vi "SW_Generate_Segmented_Plot_v2.vi"(0 "Draw Area Size":cluster{"Width":dbl, "Height":dbl}={"Width"=480.0, "Height"=480.0}, 1 "Input cluster of parameters":T1={"Amount of border segments"=8, "Border segments starting angle"=0, "Amount of midfield segments"=4, "Midfield segments starting angle"=0, "Midfield segments outer radius, mm"=60, "Amount of central segments"=1, "Center segment outer radius, mm"=30}, 2 "Diameter of the cage, mm":u16(knob)=180 scale=20.0..250.0, 3 "R-gap between segments, mm":u8=10, 4 "Colors array for outer segments":u32[](array[numeric])=[14102567, 16625249, 14742520, 7646673, 16018755, 16703632, 11262441, 4552116], 5 "Error In":errorcluster, 6 "Regions to mark":u16[](array[numeric]), 7 "Colors array for midfield segments":u32[](array[numeric])=[8073876, 10935200, 34871, 12756431], 9 "Color for central segment":u32=16777113) -> (12 "No zones Display output":picture, 14 "Zones Display output":picture, 15 "Actual parameters output":T4, 16 "Array of the segment to color correspondences":u32[][](array[numeric]), 17 "Array of the pixel to color correspondences":u32[][](array[numeric]), 18 "Pixels per mm":dbl=2.533333333333333, 19 "Error Out":errorcluster)   [LabVIEW 2018]
panel:
  out "Fonts scale factor":dbl
  out "Coordinates of the center of the image":T2
  out "Center segments outer radius, pix":dbl
  out "Midfield segments outer radius, pix":dbl
  out "Bounding rectangle of the midfield segments":T3
  out "Bounding rectangle for outer segments":T3
  in  "Fill color for no segments image":u32(colorbox)=6316128
  out "Radius of displayed outer segments, pix":dbl=228.0
  in  "Background color":u32(colorbox)=13816530
  in  "Zones Display input":picture
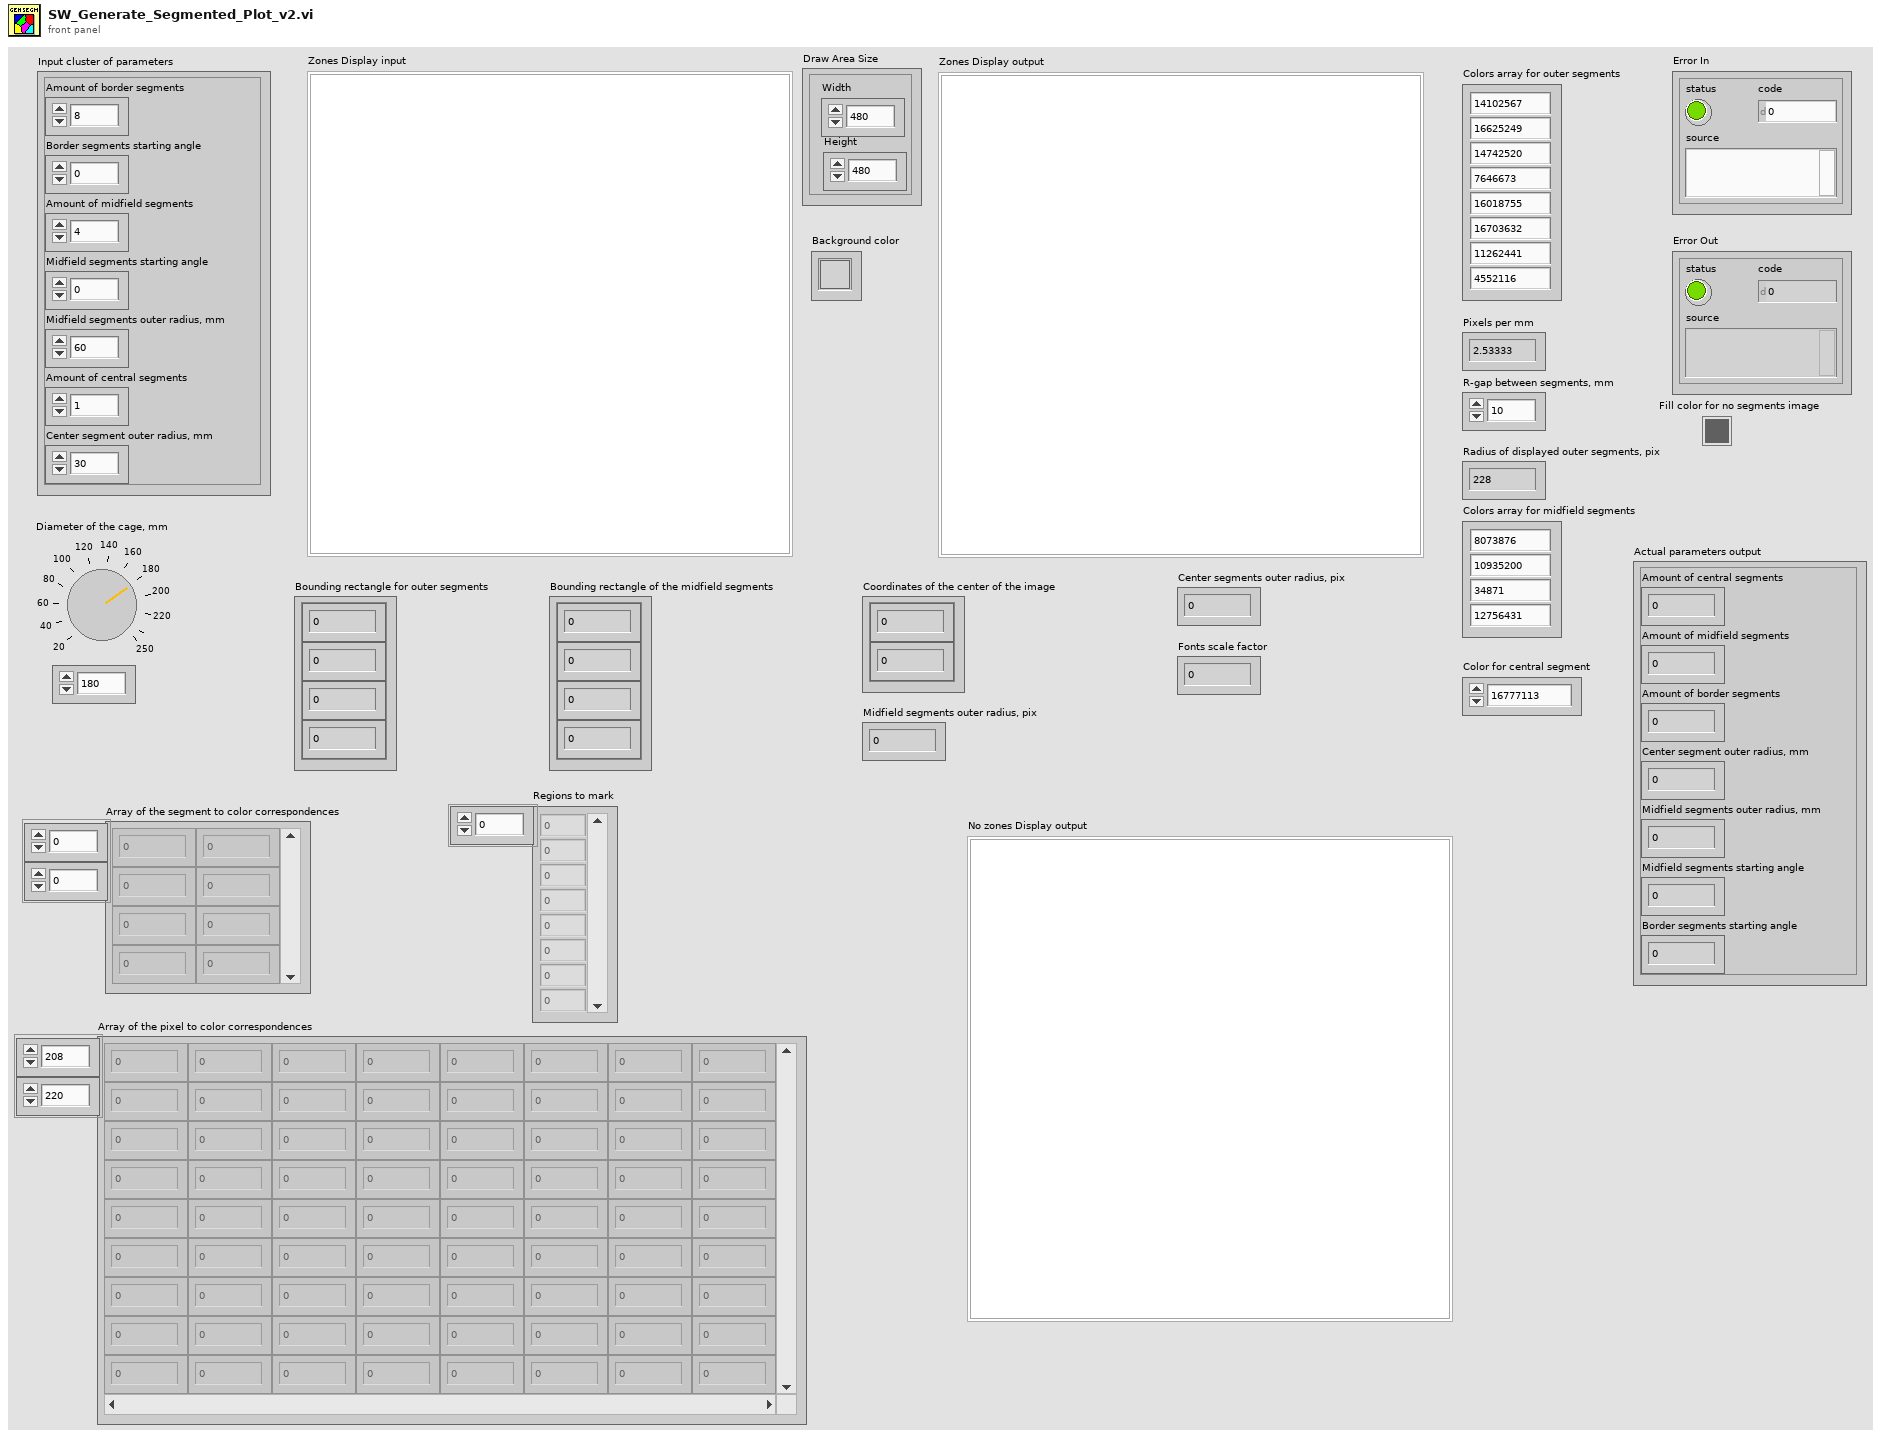
[diagram p1: front panel]
types:
  T1 = cluster{"Amount of border segments":u8, "Border segments starting angle":i16, "Amount of midfield segments":u8, "Midfield segments starting angle":i16, "Midfield segments outer radius, mm":u16, "Amount of central segments":u8, "Center segment outer radius, mm":u16}
  T2 = cluster{"Numeric Control":dbl, "Numeric Control":dbl}
  T3 = cluster{"Numeric Control":dbl, "Numeric Control":dbl, "Numeric Control":dbl, "Numeric Control":dbl}
  T4 = cluster{"Amount of central segments":u8, "Amount of midfield segments":u8, "Amount of border segments":u8, "Center segment outer radius, mm":u16, "Midfield segments outer radius, mm":u16, "Midfield segments starting angle":i16, "Border segments starting angle":i16}
  T5 = enum16{"User-specified Font", "Application Font", "System Font", "Dialog Font"}
  T6 = cluster{"horizontal":enum16{"left", "center", "right"}, "vertical":enum16{"top", "center", "bottom"}}
  T7 = cluster{"Width":u16, "Style":enum32{"Solid", "Dash", "Dot", "DashDot", "DashDotDot"}}
  T8 = cluster{"Amount of central segments":u8, "Amount of midfield segments":u8, "Amount of border segments":u8, u16, u16, i16, i16}
  T9 = typedef "imagedata.ctl" = cluster{"image type":i32, "image depth":i32, "image":u8[], "mask":u8[], "colors":u32[], "Rectangle":cluster{"left":i16, "top":i16, "right":i16, "bottom":i16}}
  T10 = cluster{"left":i16, "top":i16, "right":i16, "bottom":i16}
  T11 = cluster{"image[0]":u8, "image[1]":u8, "image[2]":u8}
  T12 = cluster{"Font Name:":string, "Size":i16, "Strikeout?":bool, "Italic?":bool, "Underline?":bool, "Outline?":bool, "Shadow?":bool, "Bold?":bool}
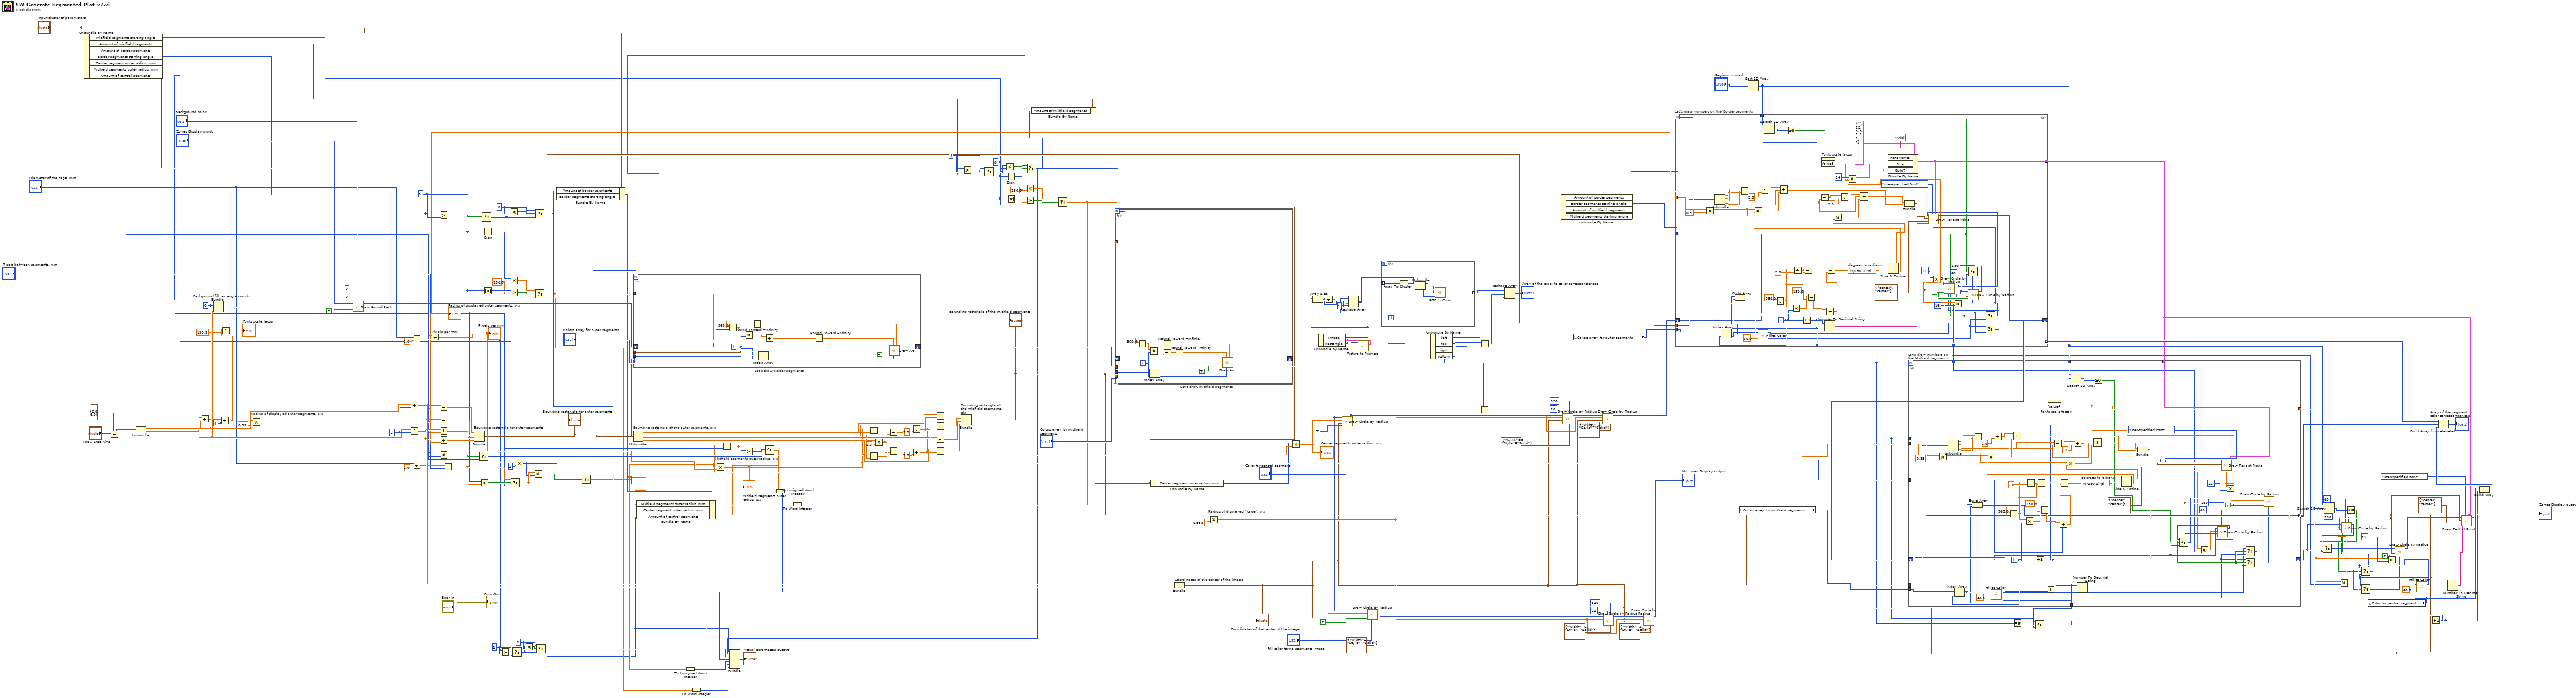
[diagram p0: block diagram]
diagram:
  w66 = 3 ("dimension size")
  w14 = TRUE ("fill?(F)")
  w150 = 180.0 ("y")
  w156 = u8 1 ("y")
  w153 = u8 1 ("y")
  w157 = u8 4 ("y")
  w160 = u8 0 ("y")
  w180 = u8 0 ("y")
  w182 = u8 8 ("y")
  w185 = 180.0 ("y")
  w194 = u32 2 ("y")
  w196 = 0
  n1 = Unbundle By Name("Input cluster of parameters") -> ("Midfield segments starting angle"=w37:i16, "Amount of midfield segments"=w36:u8, "Amount of border segments"=w35:u8, "Border segments starting angle"=w34:i16, "Center segment outer radius, mm"=w33:u16, "Midfield segments outer radius, mm"=w32:u16, "Amount of central segments"=w31:u8)
  n2 = Subtract(x="Draw Area Size", y=cluster{"Width":dbl, "Height":dbl} {"Width"=6.0, "Height"=6.0}) -> (x-y=w91:cluster{"Width":dbl, "Height":dbl})
  n3 = Unbundle(w91) -> ("Width"=w192:dbl, "Height"=w193:dbl)
  n4 = Add(x=w193, y=w192) -> (x+y=w191:dbl)
  n5 = Bundle "Background fill rectangle coords"(w196, w196, "Width"=w192, "Height"=w193) -> (w178:cluster{i32, i32, "Width":dbl, "Height":dbl})  [unwired: 1 in]
  n6 = Divide(x=w191, y=u32 4) -> (x/y=w30:dbl)
  n7 = Divide(x=w30, y=199.5) -> (x/y=→"Fonts scale factor":dbl)
  n8 = Multiply "Radius of displayed outer segments, pix"(x=w30, y=0.95) -> (x*y=w78:dbl)
  "Radius of displayed outer segments, pix" <- w78
  n9 = call <vilib>:"Draw Round Rect.vi"("picture"="Zones Display input", "oval width"=i16 0, "rect"=w178, "fill?(F)"=TRUE, "color(black)"="Background color", "oval height"=i16 0) -> ("new picture"=w177:picture)  [unwired: 3 in]
  n10 = Divide(x=w192, y=w194) -> (x/y=w176:dbl)
  n11 = Divide(x=w193, y=w194) -> (x/y=w175:dbl)
  n12 = Divide(x="Diameter of the cage, mm", y=2.0) -> (x/y=w164:dbl)
  n13 = Divide(x="Diameter of the cage, mm", y=2.0) -> (x/y=w142:dbl)
  n14 = Divide "Pixels per mm"(x=w78, y=w164) -> (x/y=w104:dbl)
  "Pixels per mm" <- w104
  n15 = Greater?(x=w35, y=w182) -> (0:w183:bool)
  n16 = Subtract(x=w176, y=w78) -> (x-y=w174:dbl)
  n17 = Subtract(x=w175, y=w78) -> (x-y=w173:dbl)
  n18 = Add(x=w176, y=w78) -> (x+y=w172:dbl)
  n19 = Add(x=w175, y=w78) -> (x+y=w171:dbl)
  n20 = Less?(x=w33, y="R-gap between segments, mm") -> (x < y?=w140:bool)
  n21 = Subtract(x=w142, y="R-gap between segments, mm") -> (x-y=w145:dbl)
  n22 = Bundle "Bounding rectangle for outer segments"(w174, w173, w172, w171) -> (w79:cluster{dbl, dbl, dbl, dbl})  [unwired: 1 in]
  "Bounding rectangle for outer segments" <- w79
  n23 = Select(t="R-gap between segments, mm", s=w140, f=w33) -> (s? t:f=w137:u16)
  n24 = Greater?(x=w32, y=w145) -> (0:w146:bool)
  n25 = Select(t=w182, s=w183, f=w35) -> (s? t:f=w179:u8)
  n26 = Sign(1:w34) -> (0:w186:i16)
  n27 = Absolute Value(x=w34) -> (abs(x)=w188:i16)
  n28 = Greater?(x=w31, y=w156) -> (0:w155:bool)
  n29 = Less?(x=w179, y=w180) -> (x < y?=w181:bool)
  n30 = Multiply(x=w186, y=w185) -> (x*y=w184:dbl)
  n31 = Greater?(x=w188, y=w185) -> (0:w187:bool)
  n32 = Select(t=w145, s=w146, f=w32) -> (s? t:f=w143:dbl)
  n33 = Select(t=w156, s=w155, f=w31) -> (s? t:f=w152:u8)
  n34 = Multiply(x="R-gap between segments, mm", y=u8 2) -> (x*y=w136:u8)
  n35 = Less?(x=w152, y=w153) -> (x < y?=w154:bool)
  n36 = Less?(x=w143, y=w136) -> (x < y?=w144:bool)
  n37 = Select(t=w180, s=w181, f=w179) -> (s? t:f=w51:u8)
  n38 = Select(t=w184, s=w187, f=w34) -> (s? t:f=w50:dbl)
  n39 = Select(t=w153, s=w154, f=w152) -> (s? t:f=w44:u8)
  n40 = Bundle By Name(cluster="Input cluster of parameters", "Amount of border segments"=w51, "Border segments starting angle"=w50) -> (w48:T1)
  n41 = Select(t=w136, s=w144, f=w143) -> (s? t:f=w46:dbl)
  n42 = for "Let's draw border segments" {
    N: w51 -> [w207]
    tunnel: w50 -> [w212]
    shift-right: [w205] -> w162
    shift-left: w177 -> [w214]
    tunnel: w79 -> [w208]
    tunnel: "Colors array for outer segments" -> [w211]
    i -> [w202]
    n43 = Divide(x=360.0, y=w207) -> (x/y=w206:dbl)
    n44 = Multiply(x=w206, y=w202) -> (x*y=w213:dbl)
    n45 = Round Toward +Infinity(x=w206) -> (ceil(x): smallest int >= x=w204:dbl)
    n46 = Index Array(array=w211, index=w202) -> (element=w201:u32)
    n47 = Add(x=w213, y=w212) -> (x+y=w209:dbl)
    n48 = Round Toward -Infinity(1:w209) -> (0:w203:dbl)
    n49 = call <vilib>:"Draw Arc.vi"("picture"=w214, "start angle[degrees]"=w203, "rect"=w208, "fill?(F)"=TRUE, "color(black)"=w201, "arc size[degrees]"=w204) -> ("new picture"=w205:picture)  [unwired: 3 in]
  }
  n50 = Unbundle "Bounding rectangle of the outer segments, pix"(w79) -> (w130:dbl, w122:dbl, w128:dbl, w121:dbl)
  n51 = To Unsigned Word Integer(number=w46) -> (unsigned 16bit integer=w109:u16)
  n52 = To Word Integer(number=w50) -> (16bit integer=w105:i16)
  n53 = Multiply "Midfield segments outer radius, pix"(x=w46, y=w104) -> (x*y=w76:dbl)
  "Midfield segments outer radius, pix" <- w76
  n54 = Subtract(x=w46, y="R-gap between segments, mm") -> (x-y=w138:dbl)
  n55 = Greater?(x=w137, y=w138) -> (0:w139:bool)
  n56 = Select(t=w138, s=w139, f=w137) -> (s? t:f=w45:dbl)
  n57 = Bundle By Name(cluster=w48, "Midfield segments outer radius, mm"=w46, "Center segment outer radius, mm"=w45, "Amount of central segments"=w44) -> (w47:T1)
  n58 = To Unsigned Word Integer(number=w45) -> (unsigned 16bit integer=w107:u16)
  n59 = Subtract(x=w128, y=w130) -> (x-y=w134:dbl)
  n60 = Subtract(x=w121, y=w122) -> (x-y=w127:dbl)
  n61 = Multiply(x=w76, y=2.0) -> (x*y=w126:dbl)
  n62 = Subtract(x=w134, y=w126) -> (x-y=w132:dbl)
  n63 = Subtract(x=w127, y=w126) -> (x-y=w124:dbl)
  n64 = Divide(x=w132, y=2.0) -> (x/y=w129:dbl)
  n65 = Divide(x=w124, y=2.0) -> (x/y=w123:dbl)
  n66 = Add(x=w130, y=w129) -> (x+y=w120:dbl)
  n67 = Add(x=w122, y=w123) -> (x+y=w118:dbl)
  n68 = Subtract(x=w128, y=w129) -> (x-y=w119:dbl)
  n69 = Subtract(x=w121, y=w123) -> (x-y=w117:dbl)
  n70 = Bundle "Bounding rectangle of the midfield segments, pix"(w120, w118, w119, w117) -> (w77:cluster{dbl, dbl, dbl, dbl})  [unwired: 1 in]
  "Bounding rectangle of the midfield segments" <- w77
  n71 = Greater?(x=w36, y=w157) -> (0:w158:bool)
  n72 = Select(t=w157, s=w158, f=w36) -> (s? t:f=w161:u8)
  n73 = Less?(x=w161, y=w160) -> (x < y?=w159:bool)
  n74 = Sign(1:w37) -> (0:w149:i16)
  n75 = Absolute Value(x=w37) -> (abs(x)=w147:i16)
  n76 = Multiply(x=w149, y=w150) -> (x*y=w151:dbl)
  n77 = Greater?(x=w147, y=w150) -> (0:w148:bool)
  n78 = Select(t=w160, s=w159, f=w161) -> (s? t:f=w49:u8)
  n79 = Bundle By Name(cluster=w47, "Amount of midfield segments"=w49) -> (w42:T1)
  n80 = Select(t=w151, s=w148, f=w37) -> (s? t:f=w108:dbl)
  n81 = To Word Integer(number=w108) -> (16bit integer=w106:i16)
  n82 = Bundle("Amount of central segments"=w44, "Amount of midfield segments"=w49, "Amount of border segments"=w51, w107, w109, w106, w105) -> (→"Actual parameters output":T8)  [unwired: 1 in]
  n83 = for "Let's draw midfield segments" {
    N: w49 -> [w221]
    shift-right: [w216] -> w97
    shift-left: w162 -> [w217]
    tunnel: w108 -> [w219]
    tunnel: w46 -> [_]
    tunnel: w77 -> [w218]
    tunnel: "Colors array for midfield segments" -> [w223]
    i -> [w220]
    n84 = Divide(x=360.0, y=w221) -> (x/y=w225:dbl)
    n85 = Multiply(x=w225, y=w220) -> (x*y=w226:dbl)
    n86 = Index Array(array=w223, index=w220) -> (element=w222:u32)
    n87 = Round Toward +Infinity(x=w225) -> (ceil(x): smallest int >= x=w228:dbl)
    n88 = Add(x=w226, y=w219) -> (x+y=w227:dbl)
    n89 = Round Toward -Infinity(1:w227) -> (0:w229:dbl)
    n90 = call <vilib>:"Draw Arc.vi"("picture"=w217, "start angle[degrees]"=w229, "rect"=w218, "fill?(F)"=TRUE, "color(black)"=w222, "arc size[degrees]"=w228) -> ("new picture"=w216:picture)  [unwired: 3 in]
  }
  n91 = Unbundle By Name(w42) -> ("Center segment outer radius, mm"=w43:u16)
  n92 = Bundle "Coordinates of the center of the image"(w176, w175) -> (w17:cluster{dbl, dbl})  [unwired: 1 in]
  "Coordinates of the center of the image" <- w17
  n93 = Multiply "Radius of displayed \"cage\", pix"(x=w30, y=0.955) -> (x*y=w93:dbl)
  n94 = Multiply(x=w43, y=w104) -> (x*y=w113:dbl)
  "Center segments outer radius, pix" <- w113
  n95 = call <vilib>:"Draw Circle by Radius.vi"("color(black)"="Color for central segment", "fill?(F)"=TRUE, "pixel center"=w17, "radius"=w113, "picture"=w97) -> ("new picture"=w70:picture)  [unwired: 6 in]
  n96 = call <vilib>:"Picture to Pixmap.vi"("picture"=w70) -> ("image data"=w69:T9)  [unwired: 9 in, 1 out]
  n97 = Unbundle By Name(w69) -> ("image"=w68:u8[], "Rectangle"=w63:T10)
  n98 = Array Size(array=w68) -> (size(s)=w67:i32)
  n99 = Divide(x=w67, y=w66) -> (x/y=w65:dbl)
  n100 = Reshape Array(w68, w65, w66) -> (w64:u8[][])
  n101 = call <vilib>:"Draw Circle by Radius.vi"("pen"=T7 {"Width"=2, "Style"=enum."Solid"}, "color(black)"="Fill color for no segments image", "fill?(F)"=TRUE, "pixel center"=w17, "radius"=w93, "picture"=w97) -> ("new picture"=w94:picture)  [unwired: 5 in]
  n102 = for {
    tunnel: w64 -> [w236] mode=indexing
    tunnel: [w231] -> w62 mode=indexing
    n103 = Array To Cluster(array=w236) -> (cluster=w235:T11)
    n104 = Unbundle(w235) -> ("image[0]"=w234:u8, "image[1]"=w233:u8, "image[2]"=w232:u8)
    n105 = call <vilib>:"RGB to Color.vi"("B"=w232, "G"=w233, "R"=w234) -> ("Color"=w231:u32)
  }
  n106 = Unbundle By Name(w63) -> ("left"=w60:i16, "top"=w57:i16, "right"=w61:i16, "bottom"=w58:i16)
  n107 = Subtract(x=w58, y=w57) -> (x-y=w56:i16)
  n108 = Subtract(x=w61, y=w60) -> (x-y=w59:i16)
  n109 = Reshape Array(w62, w59, w56) -> (→"Array of the pixel to color correspondences":u32[][])
  n110 = Unbundle By Name(w42) -> ("Amount of border segments"=w41:u8, "Border segments starting angle"=w40:i16, "Amount of midfield segments"=w5:u8, "Midfield segments starting angle"=w39:i16)
  n111 = call <vilib>:"Draw Circle by Radius.vi"("pen"=T7 {"Width"=6, "Style"=enum."Solid"}, "arc size(360)"=i16 320, "start angle(0)"=i16 20, "pixel center"=w17, "radius"=w93, "picture"=w70) -> ("new picture"=w170:picture)  [unwired: 5 in]
  n112 = local read "Colors array for outer segments"() -> (w86:u32[])
  n113 = call <vilib>:"Draw Circle by Radius.vi"("pen"=T7 {"Width"=2, "Style"=enum."Solid"}, "pixel center"=w17, "radius"=w93, "picture"=w170) -> ("new picture"=w88:picture)  [unwired: 7 in]
  n114 = call <vilib>:"Draw Circle by Radius.vi"("pen"=T7 {"Width"=6, "Style"=enum."Solid"}, "arc size(360)"=i16 320, "start angle(0)"=i16 20, "pixel center"=w17, "radius"=w93, "picture"=w94) -> ("new picture"=w98:picture)  [unwired: 5 in]
  n115 = call <vilib>:"Draw Circle by Radius.vi"("pen"=T7 {"Width"=2, "Style"=enum."Solid"}, "pixel center"=w17, "radius"=w93, "picture"=w98) -> ("new picture"=→"No zones Display output":picture)  [unwired: 7 in]
  n116 = local read "Colors array for midfield segments"() -> (w85:u32[])
  n117 = Sort 1D Array(array="Regions to mark") -> (sorted array=w21:u16[])
  n118 = for "Let's draw numbers on the Border segments" {
    N: w41 -> [w303]
    tunnel: w40 -> [w304]
    shift-right: [w283] -> w87
    shift-left: w88 -> [w246]
    tunnel: w79 -> [w298]
    tunnel: w86 -> [w271]
    tunnel: w78 -> [w268]
    tunnel: [w255] -> w2
    tunnel: [w265] -> w74 mode=indexing
    tunnel: [w257] -> w27
    tunnel: w21 -> [w256]
    tunnel: [w242] -> w1
    i -> [w270]
    w242 = 16 ("y")
    w251 = TRUE ("fill?(F)")
    n119 = Multiply(x=w268, y=0.9) -> (x*y=w267:dbl)
    n120 = Unbundle(w298) -> (w292:dbl, w285:dbl, w297:dbl, w284:dbl)
    n121 = Index Array(array=w271, index=w270) -> (element=w243:u32)
    n122 = Subtract(x=w297, y=w292) -> (x-y=w295:dbl)
    n123 = call <vilib>:"Hilite Color.vi"("Percentage(30)"=60.0, "Color In"=w243) -> ("Shadow"=w241:u32, "Hilite"=w240:u32)
    n124 = Divide(x=w295, y=2.0) -> (x/y=w293:dbl)
    n125 = Divide(x=360.0, y=w303) -> (x/y=w273:dbl)
    n126 = Multiply(x=w273, y=w270) -> (x*y=w277:dbl)
    n127 = Divide(x=w273, y=2.0) -> (x/y=w275:dbl)
    n128 = Increment(x=w270) -> (x+1=w255:i32)
    n129 = Build Array(w243, w255) -> (w265:u32[])
    n130 = Search 1D Array(1D array=w256, element=w255) -> (index of element=w254:i32)  [unwired: 1 in]
    n131 = Greater Or Equal To 0?(x=w254) -> (x >= 0?=w239:bool)
    n132 = Subtract(x=w275, y=w273) -> (x-y=w274:dbl)
    n133 = Subtract(x=w277, y=180.0) -> (x-y=w278:dbl)
    n134 = Subtract(x=w284, y=w285) -> (x-y=w287:dbl)
    n135 = property on="Fonts scale factor" class="DigNum (strict)"() -> ("Value"=w250:dbl)  [unwired: 2 in, 2 out]
    n136 = Number To Decimal String(number=w255) -> (decimal integer string=w281:string)  [unwired: 1 in]
    n137 = Add(x=w278, y=w304) -> (x+y=w301:dbl)
    n138 = Subtract(x=w274, y=w301) -> (x-y=w300:dbl)
    n139 = Divide(x=w287, y=2.0) -> (x/y=w289:dbl)
    n140 = Multiply(x=i16 14 ("Size"), y=w250) -> (x*y=w259:dbl)
    n141 = expression code="(x/180.0)*pi" "degrees to radians"(w300) -> (w299:dbl)
    n142 = Bundle By Name(cluster=T12 {"Font Name:"="", "Size"=12, "Strikeout?"=FALSE, "Italic?"=FALSE, "Underline?"=FALSE, "Outline?"=FALSE, "Shadow?"=FALSE, "Bold?"=FALSE} ("[user-specified font]"), "Font Name:"="Arial", "Size"=w259, "Bold?"=TRUE) -> (w257:T12)
    n143 = Sine & Cosine(0:w299) -> (1:w286:dbl, 2:w296:dbl)
    n144 = Multiply(x=w267, y=w296) -> (x*y=w291:dbl)
    n145 = Compound Arithmetic op=ADD(w293, w292, w291) -> (w280:dbl)
    n146 = Multiply(x=w267, y=w286) -> (x*y=w290:dbl)
    n147 = Compound Arithmetic op=ADD(w289, w285, w290) -> (w279:dbl)
    n148 = Bundle(w279, w280) -> (w252:cluster{dbl, dbl})  [unwired: 1 in]
    n149 = Multiply(x=i16 11 ("radius"), y=w250) -> (x*y=w258:dbl)
    n150 = Multiply(x=w250, y=w242) -> (x*y=w249:dbl)
    n151 = Select(t=w240, s=w239, f=w241) -> (s? t:f=w237:u32)
    n152 = call <vilib>:"Draw Circle by Radius.vi"("arc size(360)"=i16 180, "color(black)"=w237, "start angle(0)"=i16 60, "fill?(F)"=w251, "pixel center"=w252, "radius"=w249, "picture"=w246) -> ("new picture"=w253:picture)  [unwired: 4 in]
    n153 = Select(t=w253, s=w239, f=w246) -> (s? t:f=w245:picture)
    n154 = Select(t=w241, s=w239, f=w240) -> (s? t:f=w238:u32)
    n155 = call <vilib>:"Draw Circle by Radius.vi"("color(black)"=w238, "fill?(F)"=w251, "pixel center"=w252, "radius"=w258, "picture"=w245) -> ("new picture"=w244:picture)  [unwired: 6 in]
    n156 = call <vilib>:"Draw Text at Point.vi"("[user-specified font]"=w257, "text color(black)"=w237, "desired font(Application)"=T5."User-specified Font", "text"=w281, "alignment(left, top)"=T6 {"horizontal"=enum."center", "vertical"=enum."center"}, "origin"=w252, "picture"=w244) -> ("new picture"=w283:picture)  [unwired: 3 in, 1 out]
  }
  n157 = for "Let's draw numbers on the Midfield segments" {
    N: w5 -> [w369]
    tunnel: w39 -> [w370]
    shift-right: [w348] -> w19
    shift-left: w87 -> [w319]
    tunnel: w77 -> [w364]
    tunnel: w85 -> [w332]
    tunnel: w76 -> [w351]
    tunnel: w2 -> [w329]
    tunnel: [w321] -> w3
    tunnel: [w327] -> w73 mode=indexing
    tunnel: w27 -> [w324]
    tunnel: [w312] -> w16
    tunnel: w21 -> [w322]
    tunnel: w1 -> [w311]
    i -> [w331]
    w315 = TRUE ("fill?(F)")
    n158 = Multiply(x=w351, y=0.85) -> (x*y=w345:dbl)
    n159 = Unbundle(w364) -> (w358:dbl, w350:dbl, w363:dbl, w349:dbl)
    n160 = Index Array(array=w332, index=w331) -> (element=w328:u32)
    n161 = Subtract(x=w363, y=w358) -> (x-y=w361:dbl)
    n162 = call <vilib>:"Hilite Color.vi"("Percentage(30)"=60.0, "Color In"=w328) -> ("Shadow"=w308:u32, "Hilite"=w307:u32)
    n163 = Divide(x=w361, y=2.0) -> (x/y=w359:dbl)
    n164 = Divide(x=360.0, y=w369) -> (x/y=w335:dbl)
    n165 = Multiply(x=w335, y=w331) -> (x*y=w340:dbl)
    n166 = Divide(x=w335, y=2.0) -> (x/y=w337:dbl)
    n167 = Increment(x=w331) -> (x+1=w338:i32)
    n168 = Subtract(x=w337, y=w335) -> (x-y=w336:dbl)
    n169 = Subtract(x=w340, y=180.0) -> (x-y=w341:dbl)
    n170 = Add(x=w338, y=w329) -> (x+y=w321:i32)
    n171 = Build Array(w328, w321) -> (w327:u32[])
    n172 = property on="Fonts scale factor" class="DigNum (strict)"() -> ("Value"=w312:dbl)  [unwired: 2 in, 2 out]
    n173 = Subtract(x=w349, y=w350) -> (x-y=w353:dbl)
    n174 = Add(x=w341, y=w370) -> (x+y=w367:dbl)
    n175 = Subtract(x=w336, y=w367) -> (x-y=w366:dbl)
    n176 = Search 1D Array(1D array=w322, element=w321) -> (index of element=w323:i32)  [unwired: 1 in]
    n177 = Divide(x=w353, y=2.0) -> (x/y=w355:dbl)
    n178 = Number To Decimal String(number=w321) -> (decimal integer string=w346:string)  [unwired: 1 in]
    n179 = expression code="(x/180.0)*pi" "degrees to radians"(w366) -> (w365:dbl)
    n180 = Greater Or Equal To 0?(x=w323) -> (x >= 0?=w309:bool)
    n181 = Sine & Cosine(0:w365) -> (1:w352:dbl, 2:w362:dbl)
    n182 = Multiply(x=w345, y=w362) -> (x*y=w357:dbl)
    n183 = Compound Arithmetic op=ADD(w359, w358, w357) -> (w343:dbl)
    n184 = Multiply(x=w345, y=w352) -> (x*y=w356:dbl)
    n185 = Compound Arithmetic op=ADD(w355, w350, w356) -> (w342:dbl)
    n186 = Bundle(w342, w343) -> (w314:cluster{dbl, dbl})  [unwired: 1 in]
    n187 = Multiply(x=w312, y=w311) -> (x*y=w313:dbl)
    n188 = Multiply(x=w312, y=i16 11 ("radius")) -> (x*y=w325:dbl)
    n189 = Select(t=w307, s=w309, f=w308) -> (s? t:f=w306:u32)
    n190 = call <vilib>:"Draw Circle by Radius.vi"("arc size(360)"=i16 180, "color(black)"=w306, "start angle(0)"=i16 60, "fill?(F)"=w315, "pixel center"=w314, "radius"=w313, "picture"=w319) -> ("new picture"=w318:picture)  [unwired: 4 in]
    n191 = Select(t=w318, s=w309, f=w319) -> (s? t:f=w320:picture)
    n192 = Select(t=w308, s=w309, f=w307) -> (s? t:f=w310:u32)
    n193 = call <vilib>:"Draw Circle by Radius.vi"("color(black)"=w310, "fill?(F)"=w315, "pixel center"=w314, "radius"=w325, "picture"=w320) -> ("new picture"=w333:picture)  [unwired: 6 in]
    n194 = call <vilib>:"Draw Text at Point.vi"("[user-specified font]"=w324, "text color(black)"=w306, "desired font(Application)"=T5."User-specified Font", "text"=w346, "alignment(left, top)"=T6 {"horizontal"=enum."center", "vertical"=enum."center"}, "origin"=w314, "picture"=w333) -> ("new picture"=w348:picture)  [unwired: 3 in, 1 out]
  }
  n195 = Equal To 0?(x=w5) -> (x = 0?=w6:bool)
  n196 = Select(t=w2, s=w6, f=w3) -> (s? t:f=w4:i32)
  n197 = Multiply(x=w16, y=w1) -> (x*y=w15:dbl)
  n198 = local read "Color for central segment"() -> (w75:u32)
  n199 = Multiply(x=w16, y=i16 11 ("radius")) -> (x*y=w25:dbl)
  n200 = call <vilib>:"Hilite Color.vi"("Percentage(30)"=60.0, "Color In"=w75) -> ("Shadow"=w10:u32, "Hilite"=w11:u32)
  n201 = Increment(x=w4) -> (x+1=w20:i32)
  n202 = Search 1D Array(1D array=w21, element=w20) -> (index of element=w22:i32)  [unwired: 1 in]
  n203 = Greater Or Equal To 0?(x=w22) -> (x >= 0?=w9:bool)
  n204 = Select(t=w11, s=w9, f=w10) -> (s? t:f=w7:u32)
  n205 = call <vilib>:"Draw Circle by Radius.vi"("arc size(360)"=i16 180, "color(black)"=w7, "start angle(0)"=i16 60, "fill?(F)"=w14, "pixel center"=w17, "radius"=w15, "picture"=w19) -> ("new picture"=w18:picture)  [unwired: 4 in]
  n206 = Select(t=w18, s=w9, f=w19) -> (s? t:f=w23:picture)
  n207 = Select(t=w10, s=w9, f=w11) -> (s? t:f=w8:u32)
  n208 = call <vilib>:"Draw Circle by Radius.vi"("color(black)"=w8, "fill?(F)"=w14, "pixel center"=w17, "radius"=w25, "picture"=w23) -> ("new picture"=w82:picture)  [unwired: 6 in]
  n209 = Number To Decimal String(number=w20) -> (decimal integer string=w80:string)  [unwired: 1 in]
  n210 = call <vilib>:"Draw Text at Point.vi"("[user-specified font]"=w27, "text color(black)"=w7, "desired font(Application)"=T5."User-specified Font", "text"=w80, "alignment(left, top)"=T6 {"horizontal"=enum."center", "vertical"=enum."center"}, "origin"=w17, "picture"=w82) -> ("new picture"=→"Zones Display output":picture)  [unwired: 3 in, 1 out]
  n211 = Build Array(w75, w20) -> (w72:u32[])
  n212 = Build Array (concatenate)(w74, w73, w72) -> (→"Array of the segment to color correspondences":u32[][])
  "Error Out" <- "Error In"
